vi "Clear timeout error.vi"(8 "error in (no error)":errorcluster) -> (0 "error out":errorcluster)   [LabVIEW 2009]
doc: "Checks to see if a timeout error has occurred, and if so, clears the error."
uses:
  <vilib>/Utility/error.llb/DialogType.ctl
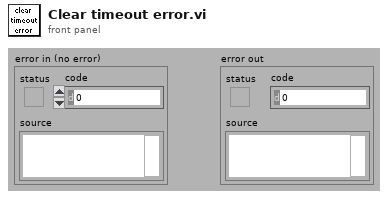
[diagram p1: front panel]
types:
  T1 = typedef "DialogType.ctl" = u16
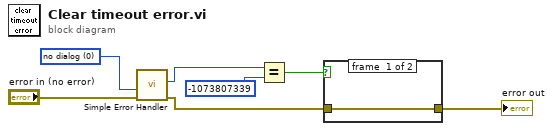
[diagram p0: block diagram]
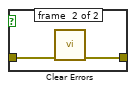
[diagram p2: hidden frame]
diagram:
  w7 = T1 0 items=["no dialog", "OK message", "continue or stop message", "OK message + warnings", "continue/stop + warnings"] ("type of dialog (OK msg:1)")
  n1 = call <vilib>:"Simple Error Handler.vi"("type of dialog (OK msg:1)"=w7, "error in (no error)"="error in (no error)") -> ("code out"=w6:i32, "error out"=w3:errorcluster)  [unwired: 6 out]
  n2 = Equal?(x=w6, y=-1073807339) -> (x = y?=w4:bool)
  n3 = case shown="True" w4 {
    tunnel: w3 -> [w8 w10]
    tunnel: [w8 w9] -> w2
    frame #0 {
    }
    frame #1 {
      n4 = call <vilib>:"Clear Errors.vi"("error in (no error)"=w10) -> ("error out"=w9:errorcluster)  [unwired: 6 out]
    }
  }
  "error out" <- w2
